vi "Config Close Inlet Outlet Step.vi"(0 "FPGA API in":refnum<class "FPGA API.lvclass">, 5 "sp [mA]":dbl, 11 "error in (no error)":errorcluster, 13 "Enum":T1(ring)) -> (4 "FPGA API out":refnum<class "FPGA API.lvclass">, 6 "sp [mA] dub":dbl, 15 "error out":errorcluster)   [LabVIEW 2019, in "FPGA API.lvclass"]
uses:
  FPGA API.lvclass
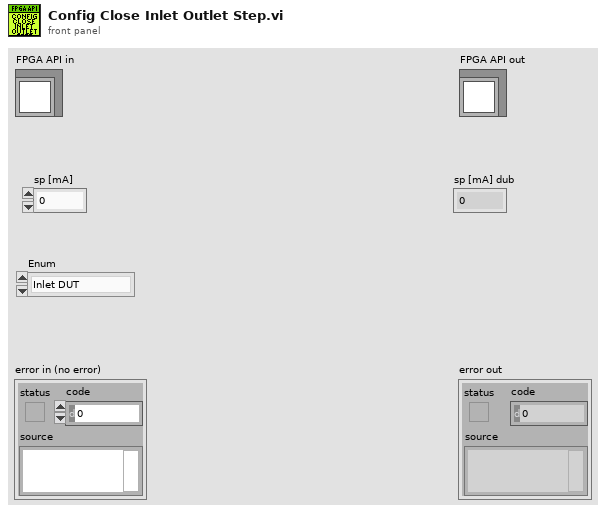
[diagram p1: front panel]
types:
  T1 = enum16{"Inlet DUT", "Outlet DUT", "StepDrive DUT", "Inlet Chamber", "Outlet Chamber", "StepDrive Chamber"}
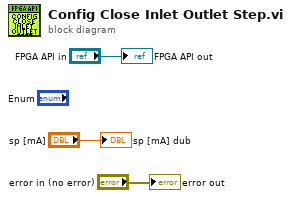
[diagram p0: block diagram]
diagram:
  "error out" <- "error in (no error)"
  "FPGA API out" <- "FPGA API in"
  "sp [mA] dub" <- "sp [mA]"
